vi "Write GratingType.vi"(8 "error in (no error)":errorcluster, 10 "GratingType":T1, 11 "SelectGrating in":refnum<class "SelectGrating.lvclass">) -> (0 "error out":errorcluster, 3 "SelectGrating out":refnum<class "SelectGrating.lvclass">)   [LabVIEW 2020, in "SelectGrating.lvclass"]
uses:
  SelectGrating.lvclass
  Typedefs/GratingType.ctl
  SelectGrating.lvclass/SelectGrating.ctl
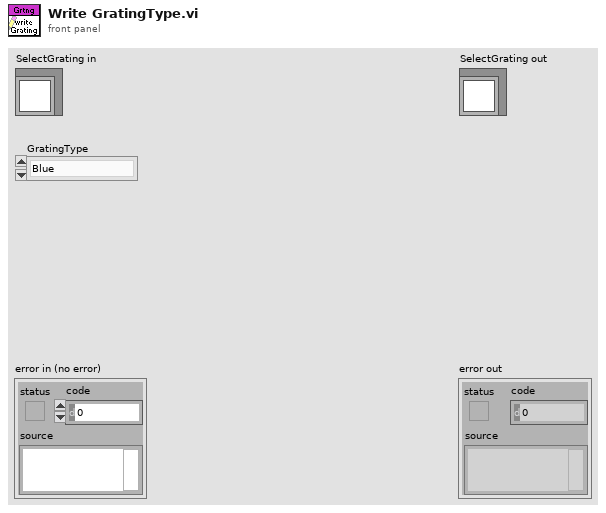
[diagram p1: front panel]
types:
  T1 = typedef "GratingType.ctl" = enum16{"Blue", "Red", "Mirror"}
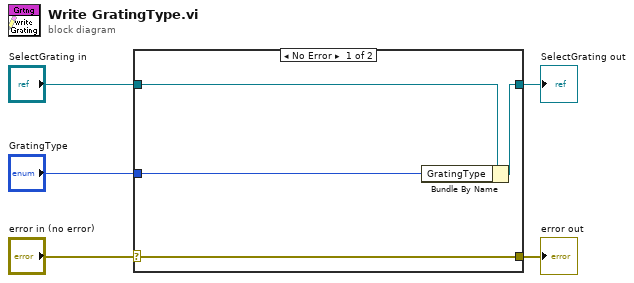
[diagram p0: block diagram]
diagram:
  n1 = case shown="No Error" "error in (no error)" {
    selector: "error in (no error)" -> [w9 w10]
    tunnel: [w9 w10] -> w4
    tunnel: [w7 w11] -> w2
    tunnel: "SelectGrating in" -> [w8 w11]
    tunnel: "GratingType" -> [w6 _]
    frame No Error {
      n2 = Bundle By Name(cluster=w8, "GratingType"=w6) -> (w7:refnum<class "SelectGrating.lvclass">)
    }
    frame Error {
    }
  }
  "error out" <- w4
  "SelectGrating out" <- w2
